vi "CTL_SelectSpec.vi"(8 "Spec RNG In":T1[](array[typedef]), 9 "Test Index":i32, 10 "Level":dbl, 11 "FullConfig":T3={"Bench Params"={"Relative Root Name"="", "Values"={"Step Levels"=0.0, "Resistor Tolerence"=0.0, "Sample Rate"=0.0, "Resistor"=0.0, "Wait Time"=0.0}, "Report Template path"=path "$ReportFiles/ReportTemplate_03.xlsx", "Test Type"="", "Config File Name"="", "Config 2 Use"=""}, "Test Params"=[], "Pump Params"={"Empty Inches"=0.0, "Full Inches"=0.0, "RNG_SLOW"=0.0, "RNG_CREEP"=0.0, "RNG_STOP "=0.0, "VISA resource name"="", "SPD_SLOW"=0, "SPD_CREEP"=0, "SPD_FAST"=0, "Zero template"=path "", "zero  Settle sec"=0, "Laser Slope"=0.0, "Laser Offset"=0.0, "Sim Fill Rate"=0.0, "Cal Date"="", "Cal Technician"=""}, "DataQ Params"={"Visa Name"="", "Num Chan"=0, "Cal Coef"=[], "Scale "=0, "Cal Date"="", "Cal Technicain"=""}, "Pump Control Ref"={"Fill "=refnum, "Drain"=refnum, "Level PV"=refnum, "Pump Speed"=refnum, "Run Test"=refnum, "Sim"=refnum, "Jog"=refnum, "Level SP"=refnum}, "Bench Status"={"Pump Status"=refnum, "Instrumnet\n Status"=refnum}} {"Pump Params"."Sim Fill Rate" format="%.3f"; "Pump Params"."Laser Offset" format="%.3f"; "Pump Params"."Laser Slope" format="%.3f"; "Pump Params"."RNG_STOP" format="%#_13g"; "Pump Params"."RNG_CREEP" format="%#_13g"; "Pump Params"."RNG_SLOW" format="%#_13g"}) -> (3 "Spec RNG Out":T1[](array[typedef]))   [LabVIEW 2024]
uses:
  Control Definitions/Def Spec RNG.ctl
  Control Definitions/Ded LUT_Status.ctl
  Control Definitions/DEF_BenchParams.ctl
  Control Definitions/DEF_PumpCtlRefs.ctl
  Control Definitions/Def_PumpSpeed.ctl
  Control Definitions/DEF_BenchStatus.ctl
  Control Definitions/DEF_DataqParams.ctl
  Control Definitions/DEF_PumpParams.ctl
  Control Definitions/DEF_FullConfig.ctl
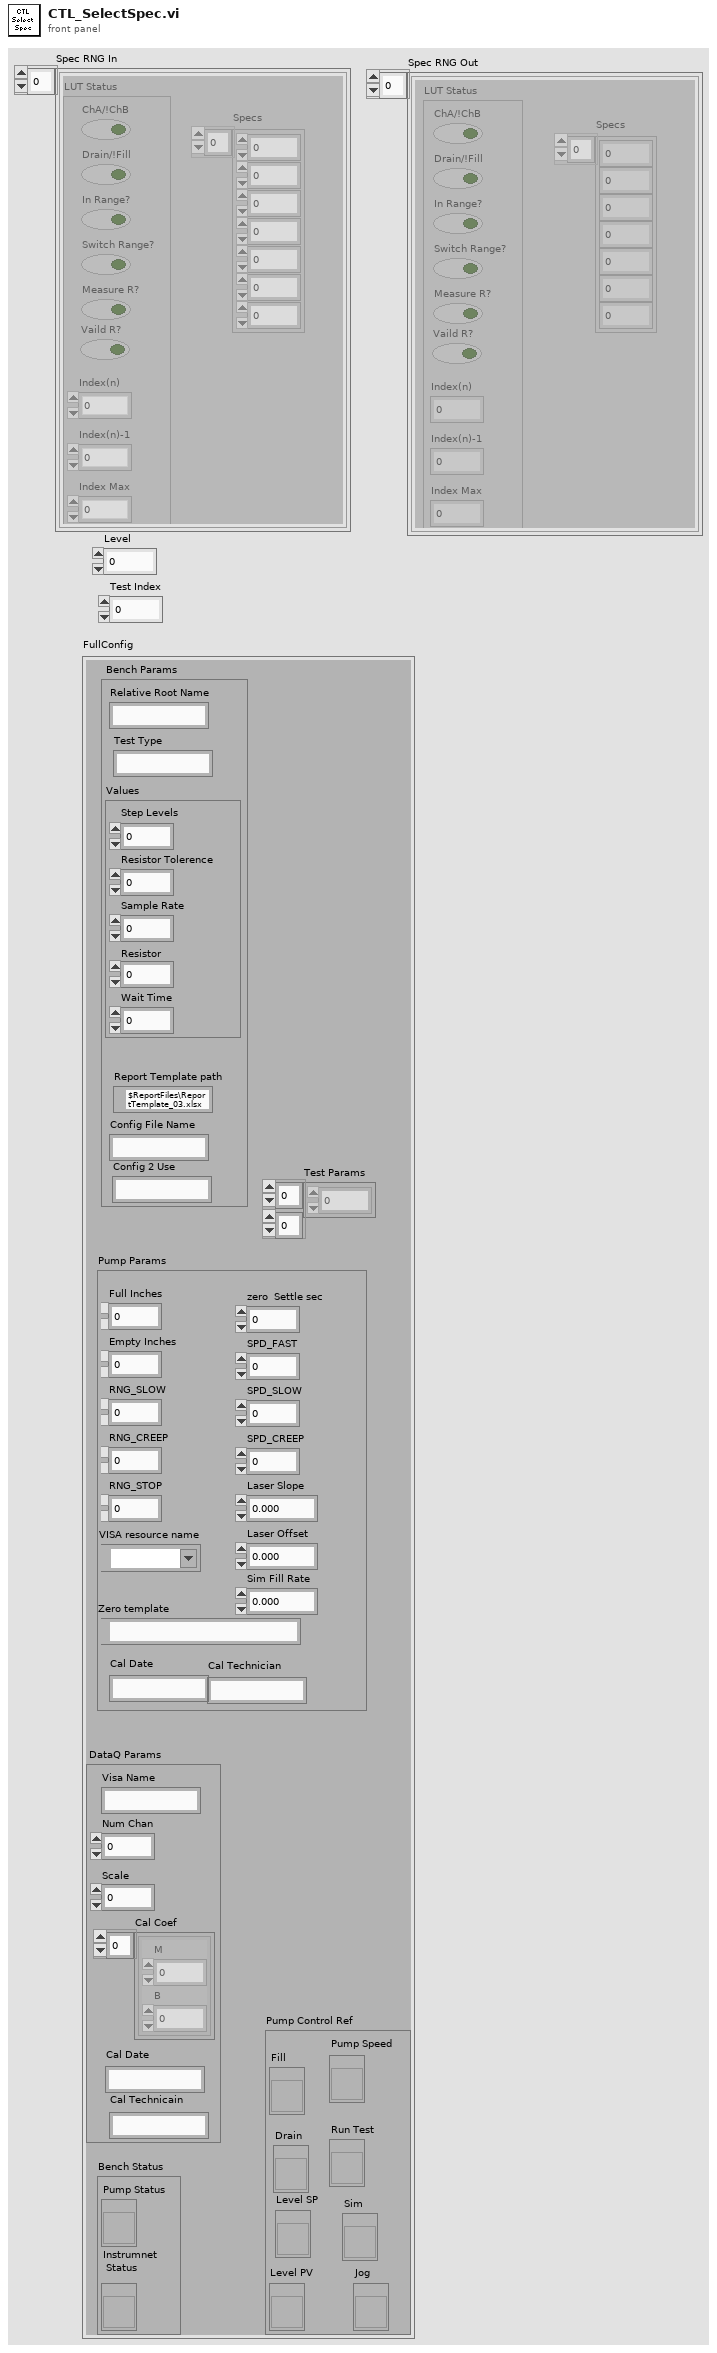
[diagram p1: front panel]
types:
  T1 = typedef "Def Spec RNG.ctl" = cluster{"Specs":dbl[], "LUT Status":T2}
  T2 = typedef "Ded LUT_Status.ctl" = cluster{"ChA/!ChB":bool, "Drain/!Fill":bool, "In Range?":bool, "Switch Range?":bool, "Measure R?":bool, "Vaild R?":bool, "Index(n)":i32, "Index(n)-1":i32, "Index Max":i32, "Index(n-1)":i32}
  T3 = typedef "DEF_FullConfig.ctl" = cluster{"Bench Params":T4, "Test Params":dbl[][], "Pump Params":T5, "DataQ Params":T6, "Pump Control Ref":T7, "Bench Status":T8}
  T4 = typedef "DEF_BenchParams.ctl" = cluster{"Relative Root Name":string, "Values":cluster{"Step Levels":dbl, "Resistor Tolerence":dbl, "Sample Rate":dbl, "Resistor":dbl, "Wait Time":dbl}, "Report Template path":path, "Test Type":string, "Config File Name":string, "Config 2 Use":string}
  T5 = typedef "DEF_PumpParams.ctl" = cluster{"Empty Inches":dbl, "Full Inches":dbl, "RNG_SLOW":dbl, "RNG_CREEP":dbl, "RNG_STOP ":dbl, "VISA resource name":refnum<visa-resource-name>, "SPD_SLOW":i32, "SPD_CREEP":i32, "SPD_FAST":i32, "Zero template":path, "zero  Settle sec":i32, "Laser Slope":sgl, "Laser Offset":sgl, "Sim Fill Rate":sgl, "Cal Date":string, "Cal Technician":string}
  T6 = typedef "DEF_DataqParams.ctl" = cluster{"Visa Name":string, "Num Chan":i32, "Cal Coef":cluster{"M":dbl, "B":dbl}[], "Scale ":i32, "Cal Date":string, "Cal Technicain":string}
  T7 = typedef "DEF_PumpCtlRefs.ctl" = cluster{"Fill ":refnum<vi>, "Drain":refnum<vi>, "Level PV":refnum<vi>, "Pump Speed":refnum<vi>, "Run Test":refnum<vi>, "Sim":refnum<vi>, "Jog":refnum<vi>, "Level SP":refnum<vi>}
  T8 = typedef "DEF_BenchStatus.ctl" = cluster{"Pump Status":refnum<vi>, "Instrumnet\n Status":refnum<vi>}
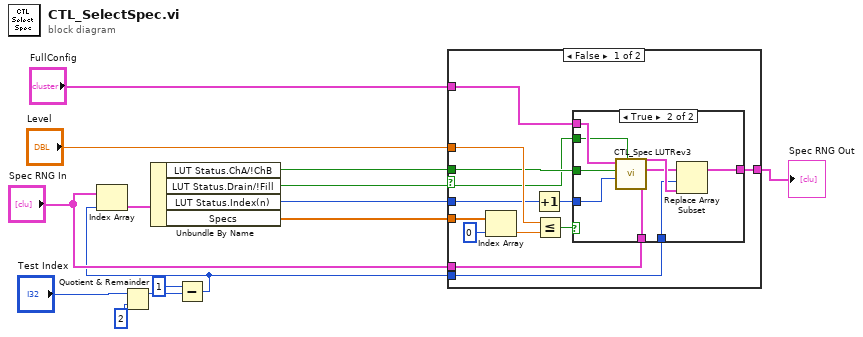
[diagram p0: block diagram]
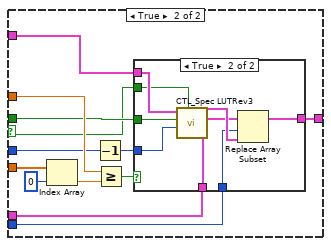
[diagram p3: hidden frame]
diagram:
  n1 = Quotient & Remainder(x="Test Index", y=2) -> (x-y*floor(x/y)=w4:i32)  [unwired: 1 out]
  n2 = Subtract(x=1, y=w4) -> (x-y=w2:i32)
  n3 = Index Array(array="Spec RNG In", index=w2) -> (element=w14:T1)
  n4 = Unbundle By Name(w14) -> ("LUT Status.ChA/!ChB"=w9:bool, "LUT Status.Drain/!Fill"=w1:bool, "LUT Status.Index(n)"=w5:i32, "Specs"=w8:dbl[])
  n5 = case shown="False" w1 {
    selector: w1 -> [w15 w37]
    tunnel: "Level" -> [w25 w47]
    tunnel: "FullConfig" -> [w24 w46]
    tunnel: w9 -> [w23 w45]
    tunnel: w8 -> [w22 w44]
    tunnel: [w21 w43] -> w7
    tunnel: "Spec RNG In" -> [w20 w42]
    tunnel: w5 -> [w17 w39]
    tunnel: w2 -> [w16 w38]
    frame False {
      n6 = Index Array(array=w22, index=0) -> (element=w26:dbl)
      n7 = Increment(x=w17) -> (x+1=w18:i32)
      n8 = Less Or Equal?(x=w25, y=w26) -> (x <= y?=w19:bool)
      n9 = case shown="True" w19 {
        tunnel: w24 -> [_ w36]
        tunnel: w23 -> [_ w35]
        tunnel: w18 -> [_ w34]
        tunnel: [w28 w32] -> w21
        tunnel: w16 -> [_ w31]
        tunnel: w20 -> [w28 w30]
        tunnel: w15 -> [_ w29]
        frame False {
        }
        frame True {
          n10 = call "CTL_Spec LUTRev3.vi"("Drain!Fill"=w29, "Index"=w34, "ChA/!ChB"=w35, "FullConfig"=w36) -> ("Spec Range Out"=w33:T1)  [unwired: 4 in, 3 out]
          n11 = Replace Array Subset(array=w30, new element=w33, index=w31) -> (w32:T1[])
        }
      }
    }
    frame True {
      n12 = Index Array(array=w44, index=0) -> (element=w48:dbl)
      n13 = Decrement(x=w39) -> (x-1=w40:i32)
      n14 = Greater Or Equal?(x=w47, y=w48) -> (x >= y?=w41:bool)
      n15 = case shown="True" w41 {
        tunnel: w46 -> [_ w58]
        tunnel: w45 -> [_ w57]
        tunnel: w40 -> [_ w56]
        tunnel: [w50 w54] -> w43
        tunnel: w38 -> [_ w53]
        tunnel: w42 -> [w50 w52]
        tunnel: w37 -> [_ w51]
        frame False {
        }
        frame True {
          n16 = call "CTL_Spec LUTRev3.vi"("Drain!Fill"=w51, "Index"=w56, "ChA/!ChB"=w57, "FullConfig"=w58) -> ("Spec Range Out"=w55:T1)  [unwired: 4 in, 3 out]
          n17 = Replace Array Subset(array=w52, new element=w55, index=w53) -> (w54:T1[])
        }
      }
    }
  }
  "Spec RNG Out" <- w7
